vi "Clear-object.vi"(8 "error in (no error)":errorcluster, 11 "Data ref.":refnum<data-value>) -> (0 "error out":errorcluster)   [LabVIEW 2013, in "CameraVision.lvlib" / "CV-Main.lvclass"]
uses:
  CV-Main.lvclass
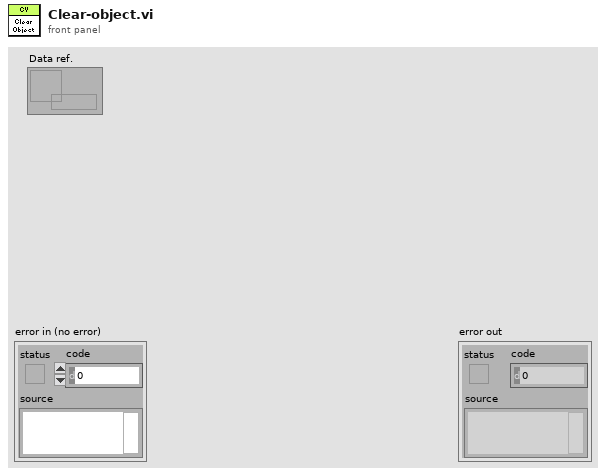
[diagram p1: front panel]
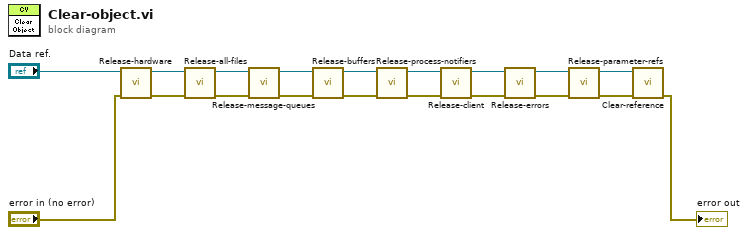
[diagram p0: block diagram]
diagram:
  n1 = call "Release-hardware.vi"("error in (no error)"="error in (no error)", "Data ref. in"="Data ref.") -> ("error out"=w13:errorcluster, "Data ref."=w17:refnum<data-value>)  [unwired: 8 in]
  n2 = call "Release-all-files.vi"("error in (no error)"=w13, "Data ref. in"=w17) -> ("error out"=w12:errorcluster, "Data ref."=w11:refnum<data-value>)  [unwired: 7 in, 1 out]
  n3 = call "Release-message-queues.vi"("error in"=w12, "Data ref. in"=w11) -> ("error IO"=w9:errorcluster, "Data ref."=w10:refnum<data-value>)  [unwired: 8 in]
  n4 = call "Release-buffers.vi"("error in"=w9, "Data ref. in"=w10) -> ("error IO"=w7:errorcluster, "Data ref."=w8:refnum<data-value>)  [unwired: 7 in, 1 out]
  n5 = call "Release-process-notifiers.vi"("error in (no error)"=w7, "Data ref. in"=w8) -> ("error out"=w16:errorcluster, "Data ref."=w6:refnum<data-value>)  [unwired: 8 in]
  n6 = call "Release-client.vi"("error in (no error)"=w16, "Data ref. in"=w6) -> ("error out"=w1:errorcluster, "Data ref."=w4:refnum<data-value>)  [unwired: 8 in]
  n7 = call "Release-errors.vi"("error in (no error)"=w1, "Data ref. in"=w4) -> ("error out"=w2:errorcluster, "Data ref."=w3:refnum<data-value>)  [unwired: 8 in]
  n8 = call "Release-parameter-refs.vi"("error in (no error)"=w2, "Data ref. in"=w3) -> ("error out"=w18:errorcluster, "Data ref."=w19:refnum<data-value>)  [unwired: 8 in]
  n9 = call "Clear-reference.vi"("error in (no error)"=w18, "Data ref."=w19) -> ("error out"=→"error out":errorcluster)  [unwired: 8 in, 1 out]
